vi "Set Actor Label.vi"(8 "error in (no error)":errorcluster, 9 "Actor Label":string, 10 "Actor's Self Q":refnum<class "Message Enqueuer.lvclass">, 11 "Monitor Data in":refnum<class "Monitor Data.lvclass">) -> (0 "error out":errorcluster, 3 "Monitor Data out":refnum<class "Monitor Data.lvclass">)   [LabVIEW 2023, in "Monitored Actor.lvlib" / "Monitor Data.lvclass"]
doc: "Changes the label for the actor\n\nCopyright: MGI 2016\nAuthor: Derek Trepanier"
uses:
  Monitor Data.lvclass
  builds/Engine/Actor Framework.lvlibp/1abvi3w/vi.lib/ActorFramework/Message Enqueuer/Message Enqueuer.lvclass
  Monitor Data.lvclass/Monitor Data.ctl
  Actor Data.ctl
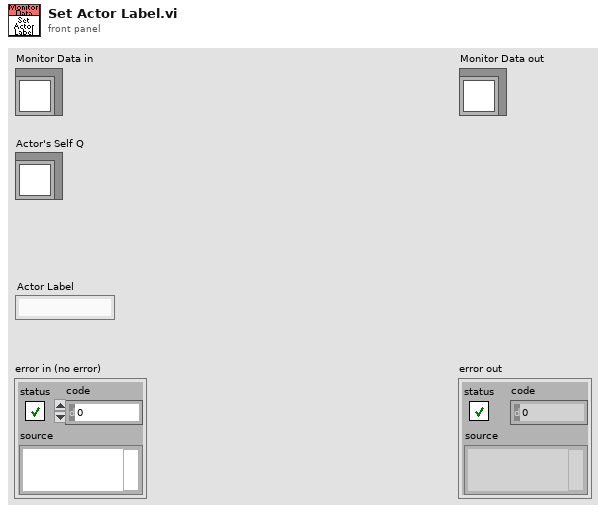
[diagram p1: front panel]
types:
  T1 = typedef "Monitored Actor.lvlib/Monitor Data.lvclass/Actor Data.ctl" = cluster{"Actor Type":string, "Actor Core VI":string, "Self":refnum<class "Message Enqueuer.lvclass">, "Caller":refnum<class "Message Enqueuer.lvclass">, "Actor Label":string, "Last Ping":dbl}
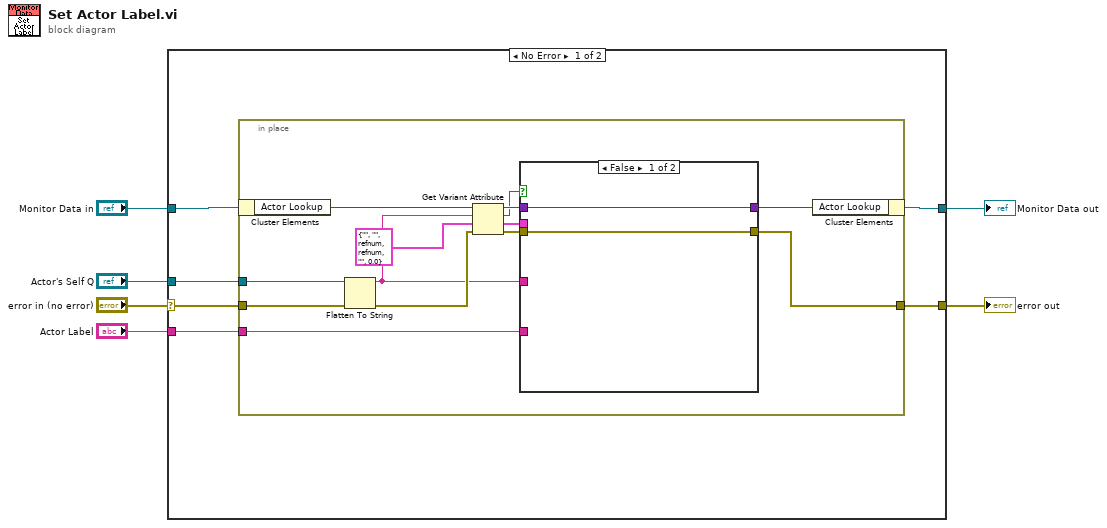
[diagram p0: block diagram]
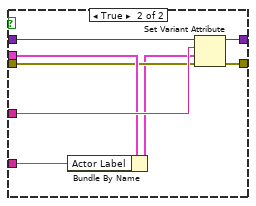
[diagram p2: hidden frame]
diagram:
  n1 = case shown="No Error" "error in (no error)" {
    selector: "error in (no error)" -> [w7 w37]
    tunnel: [w8 w37] -> w2
    tunnel: [w9 w36] -> w5
    tunnel: "Monitor Data in" -> [w10 w36]
    tunnel: "Actor's Self Q" -> [w12 _]
    tunnel: "Actor Label" -> [w11 _]
    frame No Error {
      n2 = in-place {
        in-place-border: w12 -> [w25]
        in-place-border: [w18] -> w8
        in-place-border: w11 -> [w17]
        in-place-border: w7 -> [w14]
        n3 = in-place-cluster #1(w10) -> ("Actor Lookup"=w16:variant)
        n4 = Flatten To String(anything=w25, error in (no error)=w14) -> (data string=w21:string, error out=w23:errorcluster)  [unwired: 2 in, 1 out]
        n5 = Get Variant Attribute(Variant=w16, name=w21, default value (empty Variant)=T1 {"Actor Type"="", "Actor Core VI"="", "Self"=refnum, "Caller"=refnum, "Actor Label"="", "Last Ping"=0.0} ("Actor Data"), error in=w23) -> (duplicate Variant=w22:variant, found=w13:bool, value=w20:T1, error out=w19:errorcluster)
        n6 = case shown="False" w13 {
          tunnel: w22 -> [w27 w35]
          tunnel: w21 -> [_ w34]
          tunnel: w20 -> [_ w33]
          tunnel: w19 -> [w26 w32]
          tunnel: [w26 w31] -> w18
          tunnel: w17 -> [_ w29]
          tunnel: [w27 w28] -> w15
          frame False {
          }
          frame True {
            n7 = Bundle By Name(cluster=w33, "Actor Label"=w29) -> (w30:T1)
            n8 = Set Variant Attribute(Variant=w35, name=w34, value=w30, error in=w32) -> (Variant out=w28:variant, error out=w31:errorcluster)  [unwired: 1 out]
          }
        }
        n9 = in-place-cluster #1("Actor Lookup"=w15) -> (w9:refnum<class "Monitor Data.lvclass">)
      }
    }
    frame Error {
    }
  }
  "error out" <- w2
  "Monitor Data out" <- w5
